vi "Validate Parameters.vi"(8 "error in (no error)":errorcluster, 10 "Fs (Hz)":dbl, 11 "Tone in":refnum<class "Tone.lvclass">) -> (0 "error out":errorcluster, 3 "Tone out":refnum<class "Tone.lvclass">)   [LabVIEW 2015, in "Tone.lvclass"]
uses:
  Tone.lvclass
  Tone.lvclass/Tone.ctl
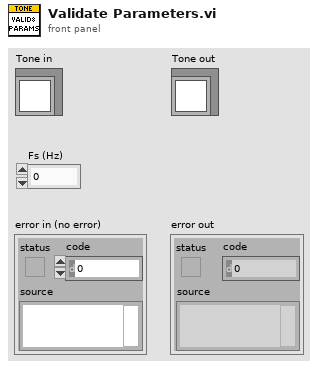
[diagram p1: front panel]
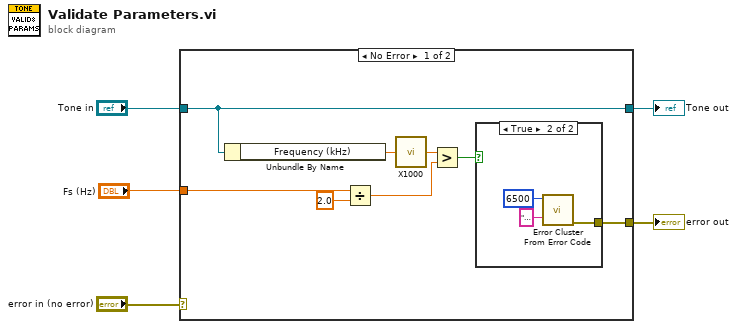
[diagram p0: block diagram]
diagram:
  n1 = case shown="No Error" "error in (no error)" {
    selector: "error in (no error)" -> [_ w18]
    tunnel: [w7 w18] -> w4
    tunnel: [w13 w17] -> w2
    tunnel: "Tone in" -> [w13 w17]
    tunnel: "Fs (Hz)" -> [w11 _]
    frame No Error {
      n2 = Unbundle By Name(w13) -> ("Frequency (kHz)"=w12:dbl)
      n3 = Divide(x=w11, y=2.0) -> (x/y=w9:dbl)
      n4 = call "X1000.vi"("X"=w12) -> ("X/1000"=w6:dbl)
      n5 = Greater?(x=w6, y=w9) -> (0:w8:bool)
      n6 = case shown="True" w8 {
        tunnel: [_ w14] -> w7
        frame False {
        }
        frame True {
          n7 = call <vilib>:"Error Cluster From Error Code.vi"("error message (\"\")"="Tone frequency must less than half the sampling rate." ("error message (\"\")"), "error code (0)"=6500) -> ("error out"=w14:errorcluster)  [unwired: 7 in]
        }
      }
    }
    frame Error {
    }
  }
  "error out" <- w4
  "Tone out" <- w2
